vi "Subscribe.vi"(8 "error in (no error)":errorcluster, 10 "Subscription Request":refnum<class "SubscriptionRequest.lvclass">, 11 "Mediator In":refnum<class "Mediator.lvclass">) -> (0 "error out":errorcluster, 3 "Mediator Out":refnum<class "Mediator.lvclass">)   [LabVIEW 2015, in "Mediator.lvlib" / "Mediator.lvclass"]
doc: "<License>\nCopyright © 2017 Composed Systems, LLC | All rights reserved\nwww.composed.io\n\nAuthor: Ethan Stern <ethan.stern@composed.io>\n\nThis software is provided \"AS IS\" WITHOUT WARRANTIES, either express or implied, AND IS FOR EDUCATIONAL PURPOSES ONLY.\n</License>"
uses:
  Mediator.lvclass
  IMediator/SubscriptionRequest/SubscriptionRequest.lvclass
  Mediator.lvclass/Mediator.ctl
  Topic Messages/Add Topic Subscriber Msg/Add Topic Subscriber Msg.lvclass/Add Topic Subscriber Msg.ctl
  <vilib>/ActorFramework/Message Enqueuer/Message Enqueuer.lvclass/Message Enqueuer.ctl
  <vilib>/ActorFramework/Message Enqueuer/Enqueue.vi
  <vilib>/ActorFramework/Message Priority Queue/Priority Enqueue.vi
  Topic Messages/Add Topic Subscriber Msg/Add Topic Subscriber Msg.lvclass
  TopicLookupTable/TopicLookupTable.lvclass
panel:
  # "Who wants it? (Unique Subscriber ID)\nWhat do they want? (Datum Name)\nWhat type are they expecting? (Variant)\nHow do they want it sent? (Transport)\nUnder what conditions? (SubscriptionPolicy)"
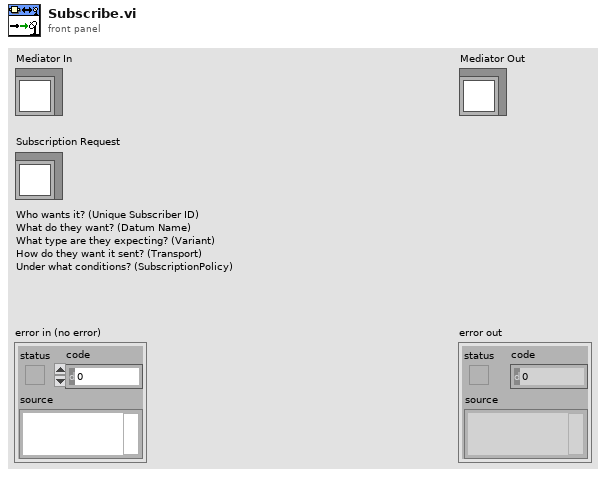
[diagram p1: front panel]
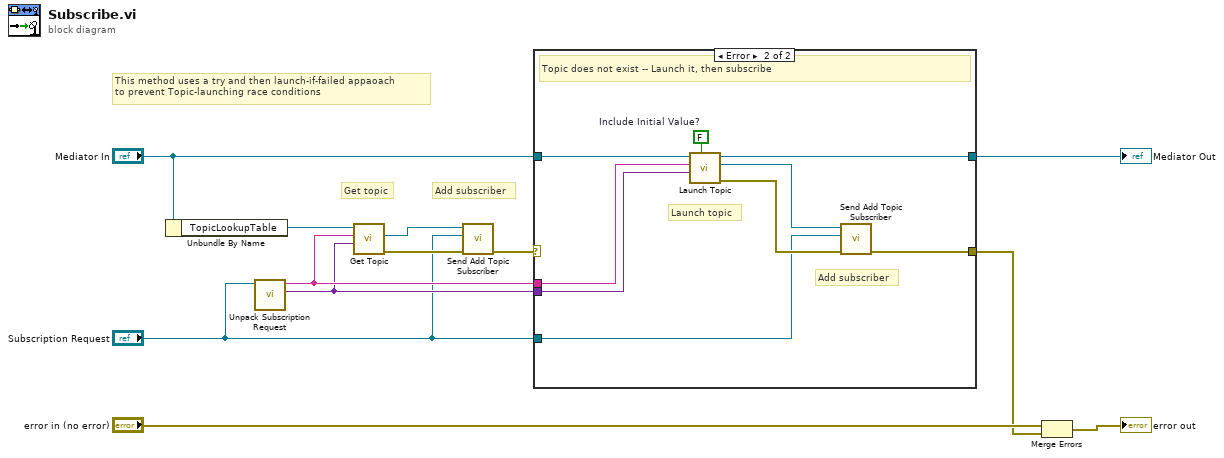
[diagram p0: block diagram]
diagram:
  # "This method uses a try and then launch-if-failed appaoach\nto prevent Topic-launching race conditions"
  # "Add subscriber"
  # "Get topic"
  n1 = Unbundle By Name("Mediator In") -> ("TopicLookupTable"=w1:refnum<data-value>)
  n2 = call "Unpack Subscription Request.vi"("SubscriptionRequest in"="Subscription Request") -> ("Type"=w4:variant, "Topic Name"=w5:string)  [unwired: 7 in, 2 out]
  n3 = call "Get Topic.vi"("Topic Type"=w4, "Topic Name"=w5, "TopicLookupTable"=w1) -> ("error out"=w6:errorcluster, "Topic Refnum"=w10:refnum<class "Message Enqueuer.lvclass">)  [unwired: 5 in, 2 out]
  n4 = call "Send Add Topic Subscriber.vi"("error in (no error)"=w6, "Subscription Request"="Subscription Request", "Message Enqueuer"=w10) -> ("error out"=w8:errorcluster)  [unwired: 7 in, 1 out]
  n5 = case shown="Error" w8 {
    selector: w8 -> [w13 _]
    tunnel: "Mediator In" -> [w14 w18]
    tunnel: [w14 w22] -> w2
    tunnel: w5 -> [_ w17]
    tunnel: w4 -> [_ w16]
    tunnel: [w13 w23] -> w7
    tunnel: "Subscription Request" -> [_ w19]
    frame No Error {
      # "Topic exists -- Subscribe OK"
    }
    frame Error {
      w15 = FALSE  # Include Initial Value?
      # "Launch topic"
      # "Add subscriber"
      # "Topic does not exist -- Launch it, then subscribe"
      n6 = call "Launch Topic.vi"("Include Initial Value? (F)"=w15, "Type"=w16, "Topic Name"=w17, "Mediator in"=w18) -> ("error out"=w20:errorcluster, "New Topic Enqueuer"=w21:refnum<class "Message Enqueuer.lvclass">, "Mediator out"=w22:refnum<class "Mediator.lvclass">)  [unwired: 5 in]
      n7 = call "Send Add Topic Subscriber.vi"("error in (no error)"=w20, "Subscription Request"=w19, "Message Enqueuer"=w21) -> ("error out"=w23:errorcluster)  [unwired: 7 in, 1 out]
    }
  }
  "Mediator Out" <- w2
  n8 = Merge Errors("error in (no error)", w7) -> (→"error out":errorcluster)
